vi "ExScanInSpectrum.vi"() -> ()   [LabVIEW 2010]
panel:
  out "Current Wavelength":dbl format="%.2f"
  out "Scanning":bool
  in  "End Wavelength":dbl=700.0 format="%.2f"
  in  "Start Wavelength":dbl format="%.2f"
  in  "Scan Speed":dbl=2000.0 min=1.0 step=1.0 format="%.2f"
  in  "Grating number":i16=1 min=1 max=100 step=1
  out "error out":errorcluster
  in  "error in (no error)":errorcluster
  # "ExScanInSpectrum.vi\nThis VI is a simple example of how to setup and scan a an InSpectrum spectrograph."
  # "NOTES:\nA properly configured spectometer .ini must be present in the LabVIEW folder for spectrograph operation.\n\nConsult the Toolkit documentation for more information on how to configure this file."
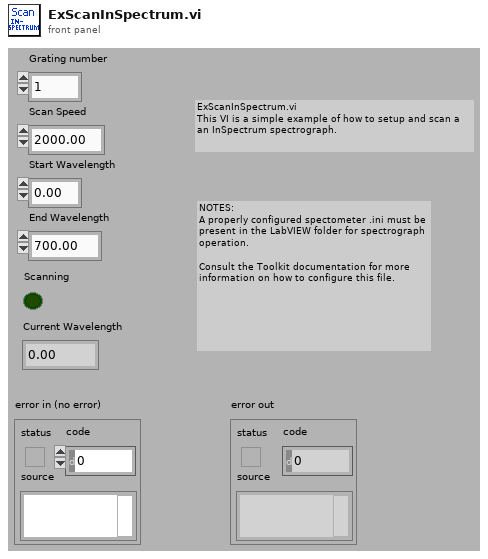
[diagram p1: front panel]
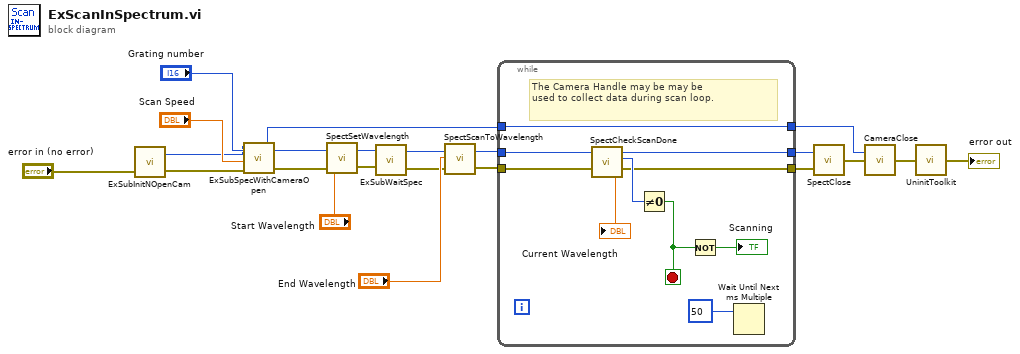
[diagram p0: block diagram]
diagram:
  n1 = call "ExSubInitNOpenCam.vi"("error in (no error)"="error in (no error)") -> ("Camera Handle"=w5:u32, "error out"=w12:errorcluster)
  n2 = call "ExSubSpecWithCameraOpen.vi"("error in (no error)"=w12, "Grating speed"="Scan Speed", "Grating number"="Grating number", "Camera Handle"=w5) -> ("error out"=w16:errorcluster, "Camera Handle"=w1:u32, "Spectrometer Handle"=w18:u32)
  n3 = call <userlib>:"SpectSetWavelength.vi"("error in"=w16, "Wavelength"="Start Wavelength", "Spectrometer Handle"=w18) -> ("error out"=w20:errorcluster, "Spectrumeter Handle"=w19:u32)
  n4 = call "ExSubWaitSpec.vi"("error in (no error)"=w20, "Spectrometer Handle"=w19) -> ("error out"=w8:errorcluster, "Spectrometer handle"=w10:u32)
  n5 = call <userlib>:"SpectScanToWavelength.vi"("error in"=w8, "Wavelength"="End Wavelength", "Spectrometer Handle"=w10) -> ("error out"=w7:errorcluster, "Spectrometer Handle"=w9:u32)
  n6 = while {
    tunnel: w9 -> [w30]
    tunnel: [w24] -> w17
    tunnel: [w25] -> w15
    tunnel: w7 -> [w31]
    tunnel: [w23] -> w2
    tunnel: w1 -> [w23]
    stop <- w27 stop-if-true
    # "The Camera Handle may be may be\nused to collect data during scan loop."
    n7 = call <userlib>:"SpectCheckScanDone.vi"("Spectrometer Handle"=w30, "error in"=w31) -> ("Spectrometer Handle"=w24:u32, "Done Flag"=w28:i16, "Wavelength"=→"Current Wavelength":dbl, "error out"=w25:errorcluster)
    n8 = Not Equal To 0?(x=w28) -> (x != 0?=w27:bool)
    n9 = Not(x=w27) -> (.not. x?=→"Scanning":bool)
    n10 = Wait Until Next ms Multiple(millisecond multiple=50) -> ()  [unwired: 1 out]
  }
  n11 = call <userlib>:"SpectClose.vi"("error in"=w15, "Spectrometer Handle"=w17) -> ("error out"=w4:errorcluster)
  n12 = call <userlib>:"CameraClose.vi"("error in"=w4, "Camera Handle"=w2) -> ("error out"=w3:errorcluster)
  n13 = call <userlib>:"UninitToolkit.vi"("error in"=w3) -> ("error out"=→"error out":errorcluster)
